vi "App.Open.vi"(8 "error in (no error)":errorcluster, 11 "State Variables":T1={"Aliases.All"=[], "Aliases.Outputs"=[], "UI.Sequence#ofColumns"=0, "SysDef.Path"=path "", "UI.SequenceRef"=refnum, "UI.StepInformationRef"=refnum, "UI.AbortRef"=refnum, "UI.GraphRef"=refnum, "UI.ViewRef"=refnum, "UI.IterationsRef"=refnum, "UI.IterationInformationRef"=refnum, "INI.Settings"={"Build Location"=path "C:/Simple Sequence Editor/SequenceRepo", "LoggingLocation"=path ""}}) -> (0 "error out":errorcluster, 3 "State Variables out":T1={"Aliases.All"=[], "Aliases.Outputs"=[], "UI.Sequence#ofColumns"=0, "SysDef.Path"=path "", "UI.SequenceRef"=refnum, "UI.StepInformationRef"=refnum, "UI.AbortRef"=refnum, "UI.GraphRef"=refnum, "UI.ViewRef"=refnum, "UI.IterationsRef"=refnum, "UI.IterationInformationRef"=refnum, "INI.Settings"={"Build Location"=path "C:/Simple Sequence Editor/SequenceRepo", "LoggingLocation"=path ""}})   [LabVIEW 2013, in "Simple Sequence Tools - Editor.lvlib"]
uses:
  Simple Sequence Tools - Editor.lvlib
  Types/StateVariables.ctl
  Shared/Types/ChannelProperties.ctl
  Shared/Types/INI.Settings
  Shared/SubVIs/Constants.vi
  Shared/Simple Sequence Tools - Shared.lvlib
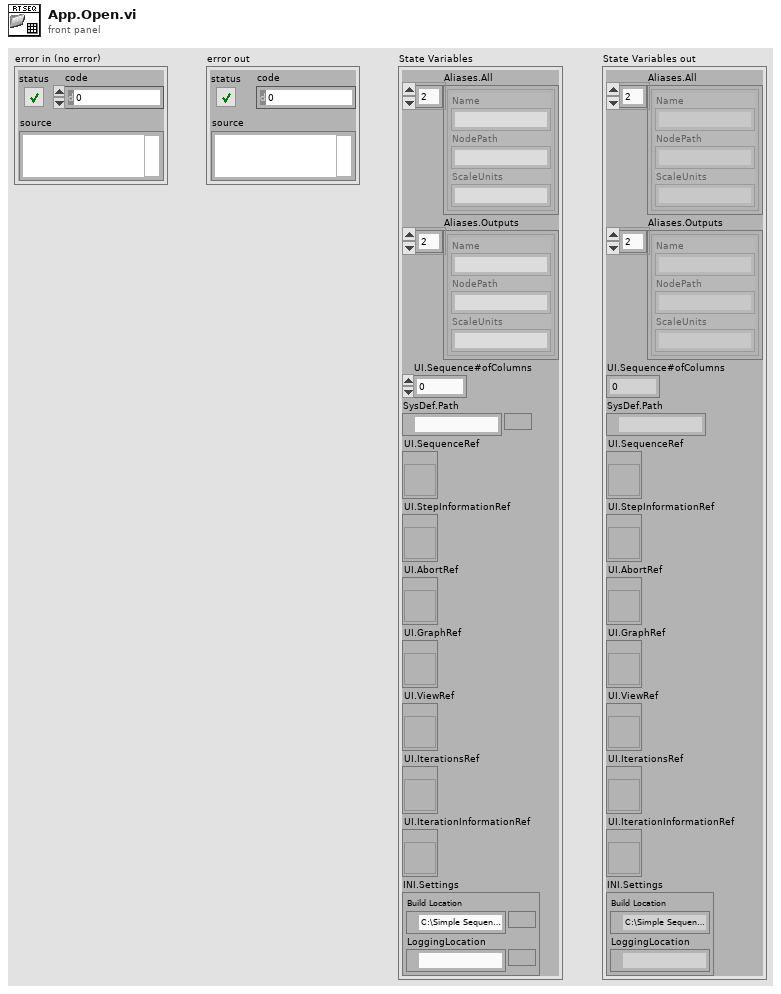
[diagram p1: front panel]
types:
  T1 = typedef "Simple Sequence Tools - Editor.lvlib/StateVariables.ctl" = cluster{"Aliases.All":T2[], "Aliases.Outputs":T2[], "UI.Sequence#ofColumns":i32, "SysDef.Path":path, "UI.SequenceRef":refnum<vi>, "UI.StepInformationRef":refnum<vi>, "UI.AbortRef":refnum<vi>, "UI.GraphRef":refnum<vi>, "UI.ViewRef":refnum<vi>, "UI.IterationsRef":refnum<vi>, "UI.IterationInformationRef":refnum<vi>, "INI.Settings":T3}
  T2 = typedef "Simple Sequence Tools - Shared.lvlib/ChannelProperties.ctl" = cluster{"Name":string, "NodePath":string, "ScaleUnits":string}
  T3 = typedef "Simple Sequence Tools - Shared.lvlib/INI.Settings" = cluster{"Build Location":path, "LoggingLocation":path}
  T4 = typedef "LVBoundsTypeDef.ctl" = cluster{"Width":u32, "Height":u32}
  T5 = typedef "Simple Sequence Tools - Shared.lvlib/Saved.Sequence.ctl" = cluster{"Output Channels":T2[], "Item Names":string[][], "Step":string, "Abort":string, "Iterations":u32, "Iteration":string}
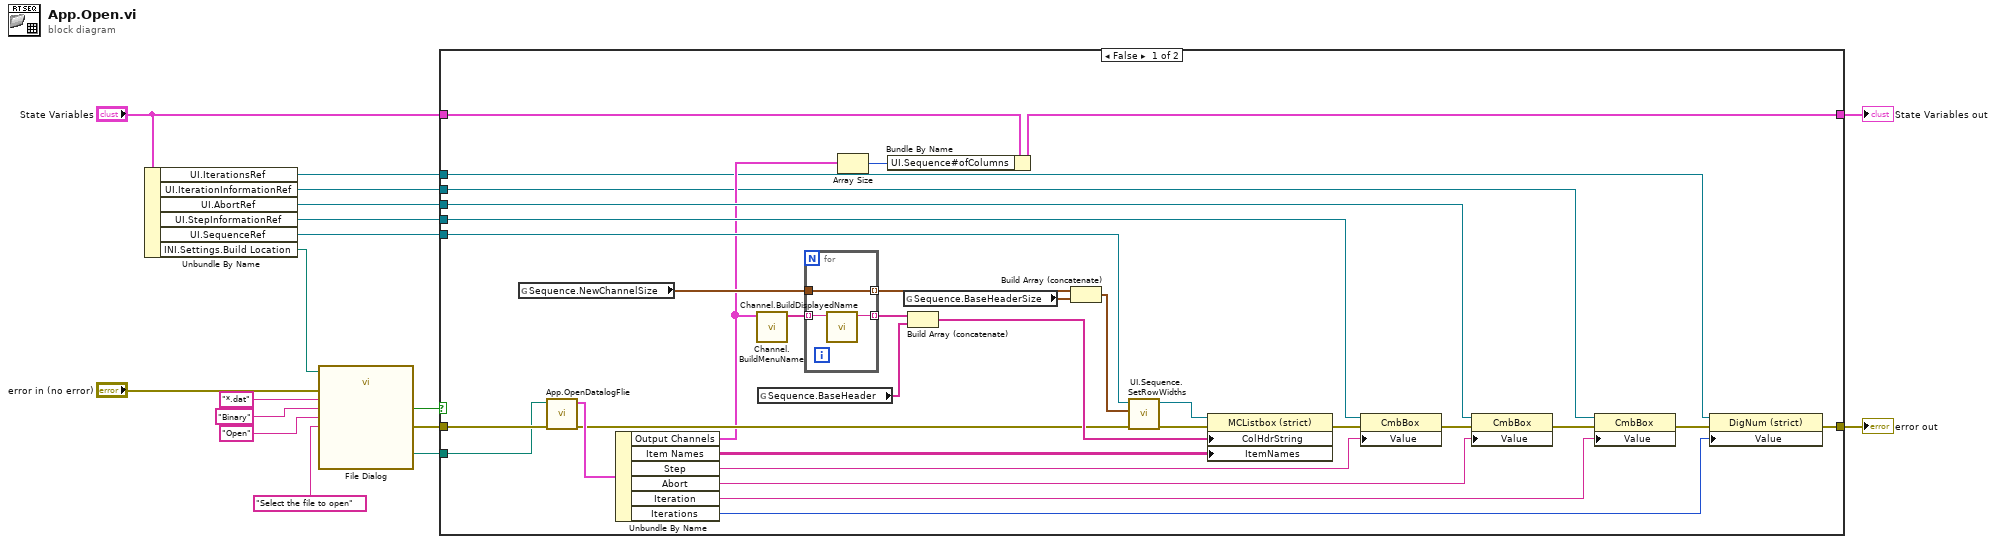
[diagram p0: block diagram]
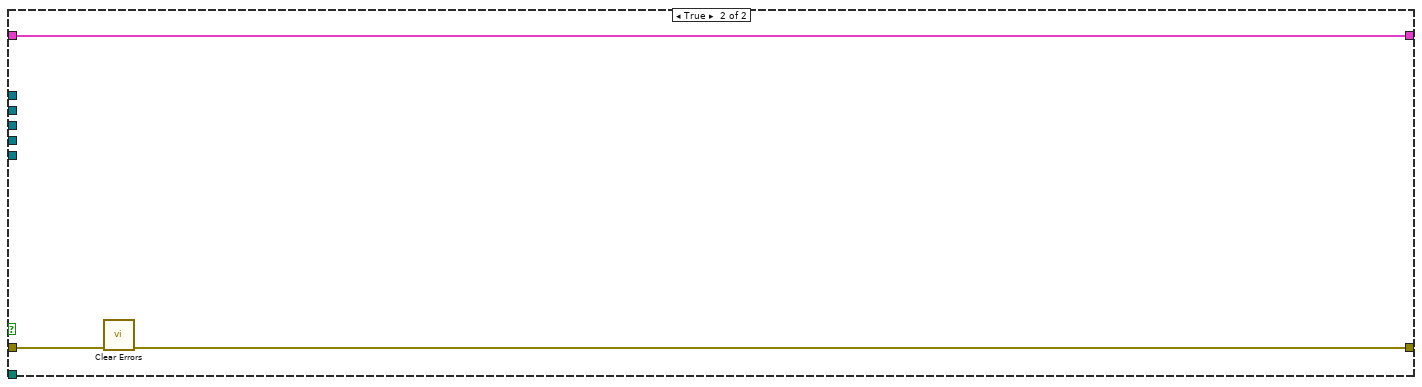
[diagram p2: hidden frame]
diagram:
  n1 = Unbundle By Name("State Variables") -> ("UI.IterationsRef"=w4:refnum<vi>, "UI.IterationInformationRef"=w3:refnum<vi>, "UI.AbortRef"=w17:refnum<vi>, "UI.StepInformationRef"=w16:refnum<vi>, "UI.SequenceRef"=w15:refnum<vi>, "INI.Settings.Build Location"=w2:path)
  n2 = call "File Dialog"("start path"=w2, "prompt"="Select the file to open", "button label"="Open", "error in"="error in (no error)", "pattern (all files)"="*.dat", "pattern label"="Binary") -> ("selected path"=w11:path, "cancelled"=w12:bool, "error out"=w7:errorcluster)  [unwired: 6 in, 1 out]
  n3 = case shown="False" w12 {
    tunnel: [w23 w55] -> w14
    tunnel: w7 -> [w50 w56]
    tunnel: w11 -> [w49 _]
    tunnel: w15 -> [w30 _]
    tunnel: w16 -> [w45 _]
    tunnel: w17 -> [w43 _]
    tunnel: "State Variables" -> [w28 w54]
    tunnel: [w25 w54] -> w5
    tunnel: w4 -> [w24 _]
    tunnel: w3 -> [w18 _]
    frame False {
      n4 = global read "Constants.vi" "Sequence.NewChannelSize"() -> (w37:T4)
      n5 = call "App.OpenDatalogFlie.vi"("error in (no error)"=w50, "selected path"=w49) -> ("error out"=w32:errorcluster, "Settings"=w48:T5)  [unwired: 8 in]
      n6 = Unbundle By Name(w48) -> ("Output Channels"=w27:T2[], "Item Names"=w47:string[][], "Step"=w44:string, "Abort"=w42:string, "Iteration"=w19:string, "Iterations"=w22:u32)
      n7 = call "Channel.BuildMenuName.vi"("Aliases"=w27) -> ("Aliases Array"=w46:string[])  [unwired: 10 in]
      n8 = global read "Constants.vi" "Sequence.BaseHeader"() -> (w38:string[])
      n9 = for {
        tunnel: w46 -> [w53] mode=indexing
        tunnel: [w52] -> w39 mode=indexing
        tunnel: [w51] -> w36 mode=indexing
        tunnel: w37 -> [w51]
        n10 = call "Channel.BuildDisplayedName.vi"("Path"=w53) -> ("Formated Path"=w52:string)  [unwired: 10 in]
      }
      n11 = Array Size(array=w27) -> (size(s)=w26:i32)
      n12 = Bundle By Name(cluster=w28, "UI.Sequence#ofColumns"=w26) -> (w25:T1)
      n13 = global read "Constants.vi" "Sequence.BaseHeaderSize"() -> (w35:T4[])
      n14 = Build Array (concatenate)(w39, w38) -> (w40:string[])
      n15 = Build Array (concatenate)(w36, w35) -> (w34:T4[])
      n16 = call "UI.Sequence.SetRowWidths.vi"("error in (no error)"=w32, "CellSize"=w34, "UI.SequenceRef"=w30) -> ("error out"=w31:errorcluster, "UI.SequenceRef"=w29:refnum<vi>)  [unwired: 7 in]
      n17 = property class="MCListbox (strict)"(reference=w29, error in=w31, "ColHdrString"=w40, "ItemNames"=w47) -> (error out=w33:errorcluster)  [unwired: 1 out]
      n18 = property class="CmbBox"(reference=w45, error in=w33, "Value"=w44) -> (error out=w41:errorcluster)  [unwired: 1 out]
      n19 = property class="CmbBox"(reference=w43, error in=w41, "Value"=w42) -> (error out=w21:errorcluster)  [unwired: 1 out]
      n20 = property class="CmbBox"(reference=w18, error in=w21, "Value"=w19) -> (error out=w20:errorcluster)  [unwired: 1 out]
      n21 = property class="DigNum (strict)"(reference=w24, error in=w20, "Value"=w22) -> (error out=w23:errorcluster)  [unwired: 1 out]
    }
    frame True {
      n22 = call <vilib>:"Clear Errors.vi"("error in (no error)"=w56) -> ("error out"=w55:errorcluster)  [unwired: 6 in]
    }
  }
  "error out" <- w14
  "State Variables out" <- w5
